vi "SwissSPAD Live_Next Image Acquisition Step.vi"(8 "Error In":errorcluster, 9 "Message in":string, 11 "SwissSPAD Live Internal Variables in":T3={"okCFrontPanelDevices Refnum"=refnum, "Bottom Device Refnum"=refnum, "Display Image"=refnum, "# Live Images"=0, "relative s"=0.0, "# Image Sets"=0, "Message"="", "Current Image Set"=0, "# Datasets in Series"=0, "Current Dataset"=0, "Live Mode"=FALSE, "Recording Mode"=FALSE, "Record Button"=refnum, "\nLive Button"=refnum, "SwissSPAD Live Gate Image Data Q Name"="SS2 Live Gate Data Q", "Discard First Image"=FALSE, "Image Information"={"Save ROI Only"=FALSE, "Left"=0, "Top"=0, "Right"=0, "Bottom"=0, "Use Current ROI"=FALSE}, "Image Binning Options"={"Use Image Binning"=FALSE, "X Bin"=1, "Y Bin"=1}, "Bottom FPGA Serial Number"="", "Detector PCB Version"=enum."SS2 PCB1", "# Acquisitions"=1, "10 bits"=FALSE, "Top FPGA Serial Number"="", "Top Device Refnum"=refnum} {"# Acquisitions" min=1; "Image Binning Options"."Y Bin" min=1; "Image Binning Options"."X Bin" min=1}) -> (0 "Error Out":errorcluster, 1 "Message out":string, 2 "SwissSPAD Live Atomic Action":T1={"SwissSPAD Q Event"=enum."Idle", "Data"=variant}, 3 "SwissSPAD Live Internal Variables out":T3={"okCFrontPanelDevices Refnum"=refnum, "Bottom Device Refnum"=refnum, "Display Image"=refnum, "# Live Images"=0, "relative s"=0.0, "# Image Sets"=0, "Message"="", "Current Image Set"=0, "# Datasets in Series"=0, "Current Dataset"=0, "Live Mode"=FALSE, "Recording Mode"=FALSE, "Record Button"=refnum, "\nLive Button"=refnum, "SwissSPAD Live Gate Image Data Q Name"="SS2 Live Gate Data Q", "Discard First Image"=FALSE, "Image Information"={"Save ROI Only"=FALSE, "Left"=0, "Top"=0, "Right"=0, "Bottom"=0, "Use Current ROI"=FALSE}, "Image Binning Options"={"Use Image Binning"=FALSE, "X Bin"=1, "Y Bin"=1}, "Bottom FPGA Serial Number"="", "Detector PCB Version"=enum."SS2 PCB1", "# Acquisitions"=1, "10 bits"=FALSE, "Top FPGA Serial Number"="", "Top Device Refnum"=refnum} {"# Acquisitions" min=1; "Image Binning Options"."Y Bin" min=1; "Image Binning Options"."X Bin" min=1})   [LabVIEW 2021]
uses:
  SwissSPAD Live_Internal Variables.ctl
  D:/UCLA Thinkpad Google Drive/LabVIEW 2021 SP1/builds/SwissSPAD Live Distribution/Opal Kelly/C# Wrapper/v5.0.2/libFrontPanel-csharp.dll
  Opal Kelly/C# Wrapper/v5.0.2/libFrontPanel-csharp.dll
  <vilib>/vision/Image Controls.llb/IMAQ Image.ctl
  SwissSPAD Live_Image ROI Information.ctl
  Phasor/Image Binning Options.ctl
  SwissSPAD Live_SSx PCB Version.ctl
  SwissSPAD Live_Q [Element].ctl
  SwissSPAD Live_Q Event List.ctl
  SwissSPAD Live_Settings List.ctl
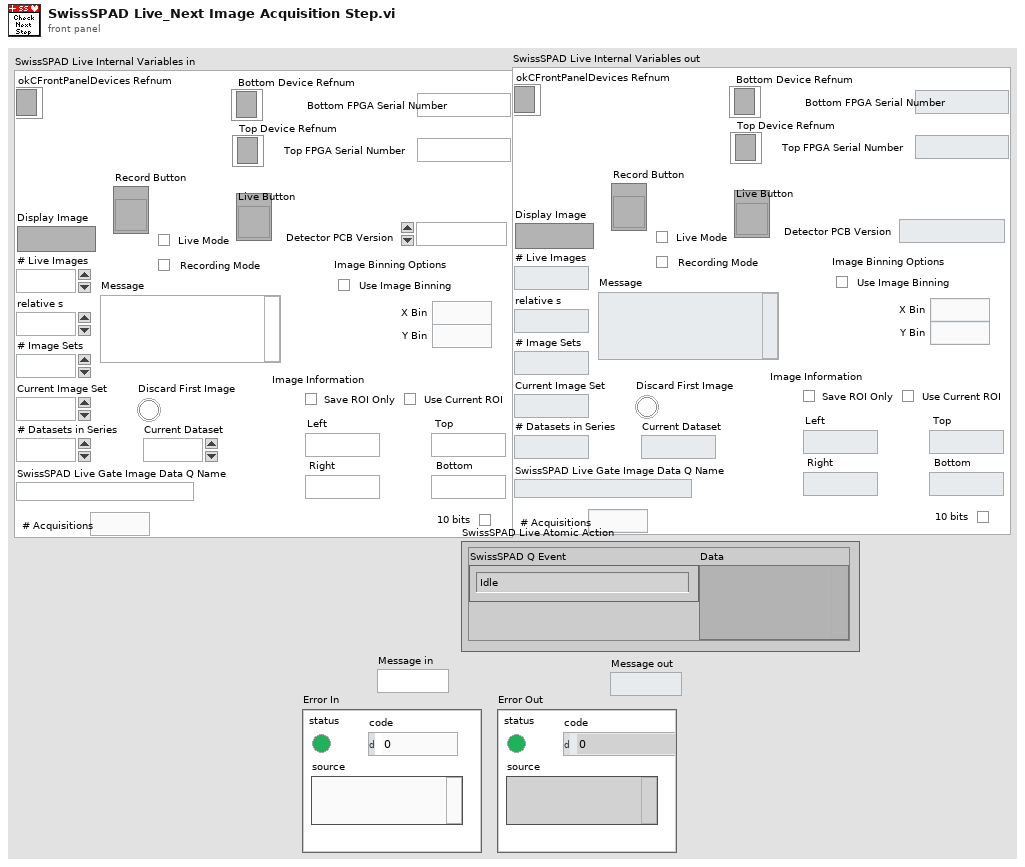
[diagram p1: front panel]
types:
  T1 = typedef "SwissSPAD Live_Q [Element].ctl" = cluster{"SwissSPAD Q Event":T2, "Data":variant}
  T2 = typedef "SwissSPAD Live_Q Event List.ctl" = enum16{"---- UI ----", "Idle", "Initialization", "Init FPGA(s)", "Init Top FPGA (deprecated)", "FPGA(s) Status", "Top FPGA Status (deprecated)", "Reset FPGA(s)", "Reset Top FPGA (deprecated)", "Refresh Display Image", "Quit", "---- DAQ ----", "Start Recording", "Start Live Acquisition", "Initialize Recording Mode", "Initialize FPGA (Live Mode)", "Get Image Set", "Get Single Image", "Update Image Display", "Stop Live Acquisition", "Stop Data Recording", "Stop Data Saving", "---- Image ----", "Copy Data to Clipboard", "Set Image Palette", "Save Displayed Image with Overlay", "Save Image Data as TIFF"}
  T3 = typedef "SwissSPAD Live_Internal Variables.ctl" = cluster{"okCFrontPanelDevices Refnum":refnum<k24>, "Bottom Device Refnum":refnum<k24>, "Display Image":T4, "# Live Images":i32, "relative s":dbl, "# Image Sets":i32, "Message":string, "Current Image Set":i32, "# Datasets in Series":i32, "Current Dataset":i32, "Live Mode":bool, "Recording Mode":bool, "Record Button":refnum<vi>, "\nLive Button":refnum<vi>, "SwissSPAD Live Gate Image Data Q Name":string, "Discard First Image":bool, "Image Information":T5, "Image Binning Options":T6, "Bottom FPGA Serial Number":string, "Detector PCB Version":T7, "# Acquisitions":u32, "10 bits":bool, "Top FPGA Serial Number":string, "Top Device Refnum":refnum<k24>}
  T4 = typedef "IMAQ Image.ctl" = refnum<image>
  T5 = typedef "SwissSPAD Live_Image ROI Information.ctl" = cluster{"Save ROI Only":bool, "Left":u16, "Top":u16, "Right":u16, "Bottom":u16, "Use Current ROI":bool}
  T6 = typedef "Image Binning Options.ctl" = cluster{"Use Image Binning":bool, "X Bin":i32, "Y Bin":i32}
  T7 = typedef "SwissSPAD Live_SSx PCB Version.ctl" = enum16{"unknown", "SS2 PCB1", "SS2 PCB2", "SS3 PCB1"}
  T8 = typedef "SwissSPAD Live_Settings List.ctl" = enum16{"FPGA:Bottom Half", "FPGA:Top Half", "FPGA:Bottom Bitfile Path", "FPGA:Top Bitfile Path", "FPGA:Bottom Bitstream Version", "FPGA:Top Bitstream Version", "FPGA:Auto Reset FPGA", "FPGA:Bottom FPGA Serial Number", "FPGA:Top FPGA Serial Number", "FPGA:Detector PCB Version", "Acquisition Parameters:Microlens", "Acquisition Parameters:SS2 DAQ Parameters", "Acquisition Parameters:Gate Configuration Array", "Acquisition Parameters:SS3 DAQ Parameters", "Acquisition Parameters:Buffer Size (# 8-bit Gates)", "File Information:File Information", "File Information:# Datasets in Series", "File Information:Scrambled File Flag", "File Information:SS3 Gate Slip Correction", "File Information:SS3 Hot Pixel Mismatch Detection", "File Information:Delay between Datasets", "File Information:Save Sum of All Gates Preview", "Image Parameters:Image ROI Information", "Image Parameters:Image Binning Options", "Image Parameters:SS3 Displayed Image", "Image Parameters:Image Display Options", "Image Parameters:Use Histogram Cursors", "Image Parameter:FPGA Data to Display", "UI Settings:Histogram Bins Number", "UI Settings:Use Image Display Options", "UI Settings:Verbose Settings", "UI Settings:Verbose Saving"}
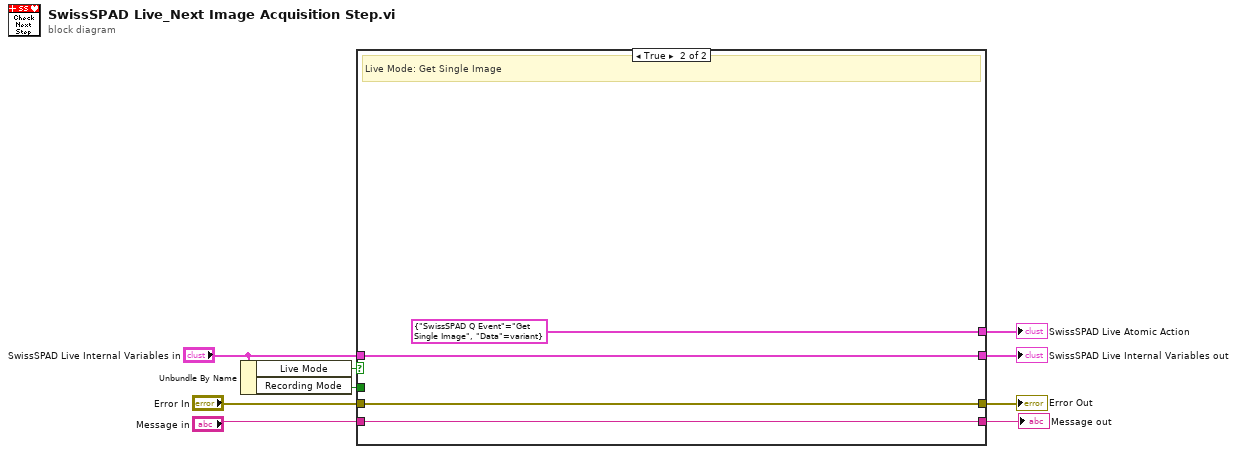
[diagram p0: block diagram]
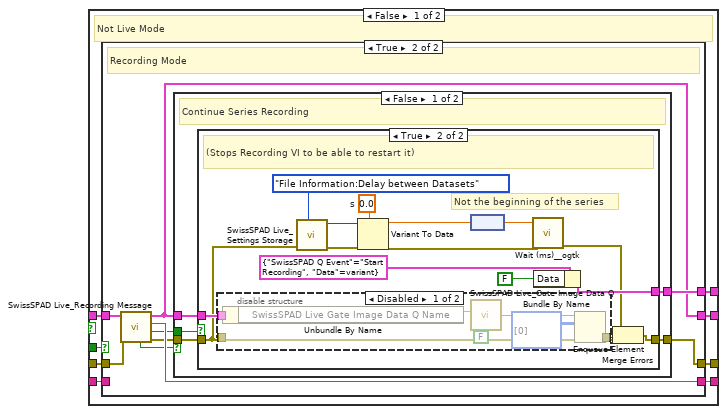
[diagram p2: hidden frame]
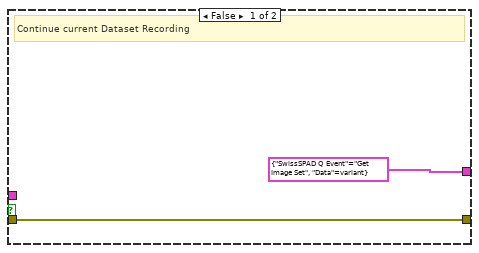
[diagram p4: hidden frame]
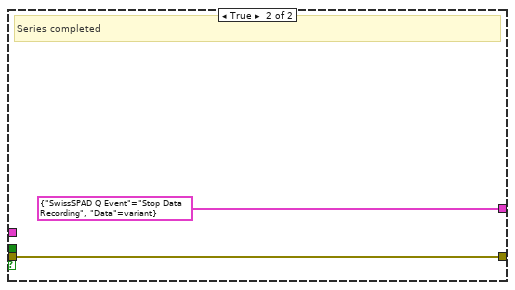
[diagram p6: hidden frame]
diagram:
  n1 = Unbundle By Name("SwissSPAD Live Internal Variables in") -> ("Live Mode"=w5:bool, "Recording Mode"=w7:bool)
  n2 = case shown="True" w5 {
    tunnel: [w12 T1 {"SwissSPAD Q Event"=enum."Get Single Image", "Data"=variant} ("SS2 Live Atomic Action")] -> w6
    tunnel: w7 -> [w13 _]
    tunnel: "SwissSPAD Live Internal Variables in" -> [w17 w63]
    tunnel: [w16 w63] -> w9
    tunnel: "Error In" -> [w15 w62]
    tunnel: [w11 w62] -> w3
    tunnel: [w14 w61] -> w2
    tunnel: "Message in" -> [w10 w61]
    frame False {
      # "Not Live Mode"
      n3 = case shown="True" w13 {
        tunnel: w17 -> [w20 w29]
        tunnel: [w20 w21] -> w16
        tunnel: w15 -> [w19 w28]
        tunnel: [w18 w27] -> w14
        tunnel: [_ w25] -> w12
        tunnel: [w19 w22] -> w11
        tunnel: w10 -> [w18 _]
        frame False {
          # "Nop"
        }
        frame True {
          # "Recording Mode"
          n4 = call "SwissSPAD Live_Recording Message.vi"("error in (no error)"=w28, "SwissSPAD Live Internal Variables"=w29) -> ("error out"=w23:errorcluster, "Current Dataset Recording Completed?"=w24:bool, "Message"=w27:string, "SwissSPAD Live Internal Variables"=w21:T3, "Dataset Series Completed?"=w26:bool)  [unwired: 5 in]
          n5 = case shown="False" w26 {
            tunnel: [w34 T1 {"SwissSPAD Q Event"=enum."Stop Data Recording", "Data"=variant} ("SS2 Live Atomic Action")] -> w25
            tunnel: w24 -> [w33 _]
            tunnel: w21 -> [w32 _]
            tunnel: w23 -> [w31 w59]
            tunnel: [w30 w59] -> w22
            frame False {
              # "Continue Series Recording"
              n6 = case shown="True" w33 {
                tunnel: [T1 {"SwissSPAD Q Event"=enum."Get Image Set", "Data"=variant} ("SS2 Live Atomic Action") w48] -> w34
                tunnel: w32 -> [_ w51]
                tunnel: w31 -> [w35 w41]
                tunnel: [w35 w40] -> w30
                frame False {
                  # "Continue current Dataset Recording"
                }
                frame True {
                  w45 = dbl[unit] 0.0  # s
                  # "Not the beginning of the series"
                  # "(Stops Recording VI to be able to restart it)"
                  n7 = disable-structure shown="Disabled" {
                    disable-tunnel: w51 -> [w56 _]
                    disable-tunnel: [w54 _] -> w49
                    disable-tunnel: w41 -> [w53 _]
                    frame Disabled {
                      n8 = Unbundle By Name(w56) -> ("SwissSPAD Live Gate Image Data Q Name"=w55:string)
                      n9 = call "SwissSPAD Live_Gate Image Data Q.vi"("create if not found? (T)"=FALSE, "SwissSPAD Live Gate Image Data Q Name"=w55) -> ("SwissSPAD Live Gate Image Data Q"=w58:refnum<queue>)  [unwired: 7 in, 2 out]
                      n10 = Enqueue Element(queue=w58, element=u8[][] [[0]], error in (no error)=w53) -> (error out=w54:errorcluster)  [unwired: 1 in, 2 out]
                    }
                    frame Enabled {
                    }
                  }
                  n11 = call "SwissSPAD Live_Settings Storage.vi"("Settings List"=SwissSPAD_Live_Settings_List."File Information:Delay between Datasets", "Error In"=w41) -> ("Error Out"=w46:errorcluster, "Variant Data out"=w37:variant)  [unwired: 8 in]
                  n12 = Variant To Data(error in=w46, type=w45, Variant=w37) -> (data=w44:dbl[unit], error out=w43:errorcluster)
                  n13 = node(w44) -> (w42:dbl)
                  n14 = call <userlib>:"Wait (ms)__ogtk.vi"("error in (no error)"=w43, "milliseconds to wait"=w42) -> ("error out"=w39:errorcluster)  [unwired: 8 in, 1 out]
                  n15 = Bundle By Name(cluster=T1 {"SwissSPAD Q Event"=enum."Start Recording", "Data"=variant} ("SS2 Live Atomic Action"), "Data"=FALSE) -> (w48:T1)
                  n16 = Merge Errors(w39, w49) -> (w40:errorcluster)
                }
              }
            }
            frame True {
              # "Series completed"
            }
          }
        }
      }
    }
    frame True {
      # "Live Mode: Get Single Image"
    }
  }
  "SwissSPAD Live Internal Variables out" <- w9
  "SwissSPAD Live Atomic Action" <- w6
  "Error Out" <- w3
  "Message out" <- w2
